vi "Channels.Inline.Data Reference to Pointer.vi"(8 "error in (no error)":errorcluster, 11 "Data Reference in":T1 format="%.0x") -> (0 "error out":errorcluster, 3 "Channel Pointer":u64)   [LabVIEW 2016, in "VeriStand Data.lvlib"]
doc: "Converts a VeriStand <B>Data Reference</B> into a <B>Channel Pointer</B> to allow for direct access of channel data."
uses:
  VeriStand Data.lvlib
  <vilib>/NI Veristand/Custom Device API/Data Reference.ctl
  <vilib>/NI Veristand/Custom Device API/Global Data Refs.vi
  <vilib>/NI Veristand/Custom Device API/Custom Device API.lvlib
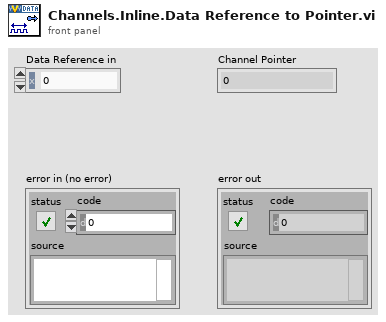
[diagram p1: front panel]
types:
  T1 = typedef "Custom Device API.lvlib/Data Reference.ctl" = i32
  T2 = typedef "Custom Device API.lvlib/Data Table Ref.ctl" = cluster{"Ptr.Beg":u64, "Ptr.End":u64}
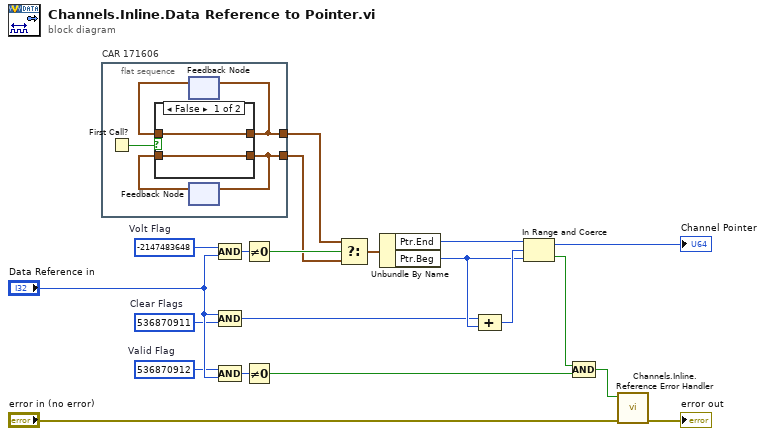
[diagram p0: block diagram]
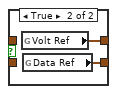
[diagram p2: hidden frame]
diagram:
  w7 = T1 536870912  # Valid Flag
  w8 = T1 536870911  # Clear Flags
  w9 = T1 -2147483648  # Volt Flag
  n1 = flat-sequence "CAR 171606" {
    tunnel: [w22] -> w6
    tunnel: [w21] -> w5
    frame #0 {
      n2 = First Call?() -> (First Call?: T/F=w25:bool)
      n3 = feedback #1() -> (w24:T2)  [unwired: 1 out]
      n4 = feedback #2() -> (w23:T2)  [unwired: 1 out]
      n5 = case shown="False" w25 {
        tunnel: [w27 w29] -> w22
        tunnel: w24 -> [w27 _]
        tunnel: [w26 w28] -> w21
        tunnel: w23 -> [w26 _]
        frame False {
        }
        frame True {
          n6 = global read "Global Data Refs.vi" "Volt Ref"() -> (w29:T2)
          n7 = global read "Global Data Refs.vi" "Data Ref"() -> (w28:T2)
        }
      }
      n8 = feedback-in #1(w22) -> ()
      n9 = feedback-in #2(w21) -> ()
    }
  }
  n10 = Compound Arithmetic op=AND(w9, "Data Reference in") -> (w15:T1)
  n11 = Compound Arithmetic op=AND("Data Reference in", w8) -> (w10:T1)
  n12 = Compound Arithmetic op=AND(w7, "Data Reference in") -> (w12:T1)
  n13 = Not Equal To 0?(x=w15) -> (x != 0?=w14:bool)
  n14 = Not Equal To 0?(x=w12) -> (x != 0?=w11:bool)
  n15 = Select(t=w6, s=w14, f=w5) -> (s? t:f=w13:T2)
  n16 = Unbundle By Name(w13) -> ("Ptr.End"=w17:u64, "Ptr.Beg"=w16:u64)
  n17 = Compound Arithmetic op=ADD(w10, w16) -> (w19:u64)
  n18 = In Range and Coerce(upper limit=w17, x=w19, lower limit=w16) -> (coerced(x)=→"Channel Pointer":u64, In Range?=w18:bool)
  n19 = Compound Arithmetic op=AND(w18, w11) -> (w1:bool)
  n20 = call "Channels.Inline.Reference Error Handler.vi"("error in (no error)"="error in (no error)", "pointer valid?"=w1) -> ("error out"=→"error out":errorcluster)  [unwired: 9 in]
